vi "Formatter.vi"(2 "error in (no error)":errorcluster, 3 "Precision (ns)":T1=enum."Nanoseconds", 4 "Variant":variant, 5 "ID":string) -> (0 "error out":errorcluster, 1 "output":string)   [LabVIEW 2023, in "Logging.lvlib"]
uses:
  Logging.lvlib
  controls/Precision.ctl
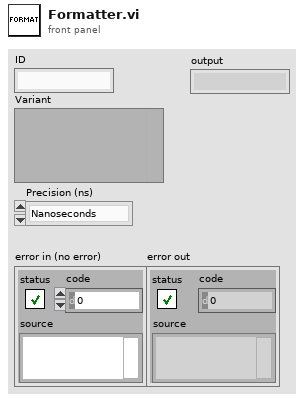
[diagram p1: front panel]
types:
  T1 = typedef "Logging.lvlib/Precision.ctl" = enum16{"Seconds", "Milliseconds", "Nanoseconds"}
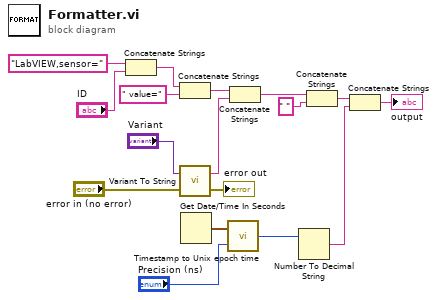
[diagram p0: block diagram]
diagram:
  n1 = Concatenate Strings("LabVIEW,sensor=" ("string"), "ID") -> (w15:string)
  n2 = Concatenate Strings(w15, " value=" ("string")) -> (w13:string)
  n3 = call "Variant To String.vi"("error in (no error)"="error in (no error)", "Variant"="Variant") -> ("error out"=→"error out":errorcluster, "String"=w12:string)
  n4 = Get Date/Time In Seconds() -> (seconds since 1Jan1904=w5:timestamp)
  n5 = call "Timestamp to Unix epoch time.vi"("Precision (ns)"="Precision (ns)", "Timestamp"=w5) -> ("Unix epoch time"=w8:u64)
  n6 = Concatenate Strings(w13, w12) -> (w9:string)
  n7 = Number To Decimal String(number=w8) -> (decimal integer string=w7:string)  [unwired: 1 in]
  n8 = Concatenate Strings(w9, " " ("string")) -> (w6:string)
  n9 = Concatenate Strings(w6, w7) -> (→"output":string)
